vi "Node - Initial Handshaking.vi"(8 "error in (no error)":errorcluster, 11 "Node Data In":T1) -> (0 "error out":errorcluster, 3 "Node Data Out":T1)   [LabVIEW 2016, in "PXImc Router.lvlib"]
uses:
  PXImc Router.lvlib
  Controls/Node Data.ctl
  <vilib>/NI Veristand/VeriStand Data/Byte Buffer/Byte Buffer.lvclass
  Controls/Node/Node - PXImc Parameters.ctl
  Controls/Node/Transfer Data.ctl
  Controls/Node/Node Ch Properties.ctl
  Controls/Data Type.ctl
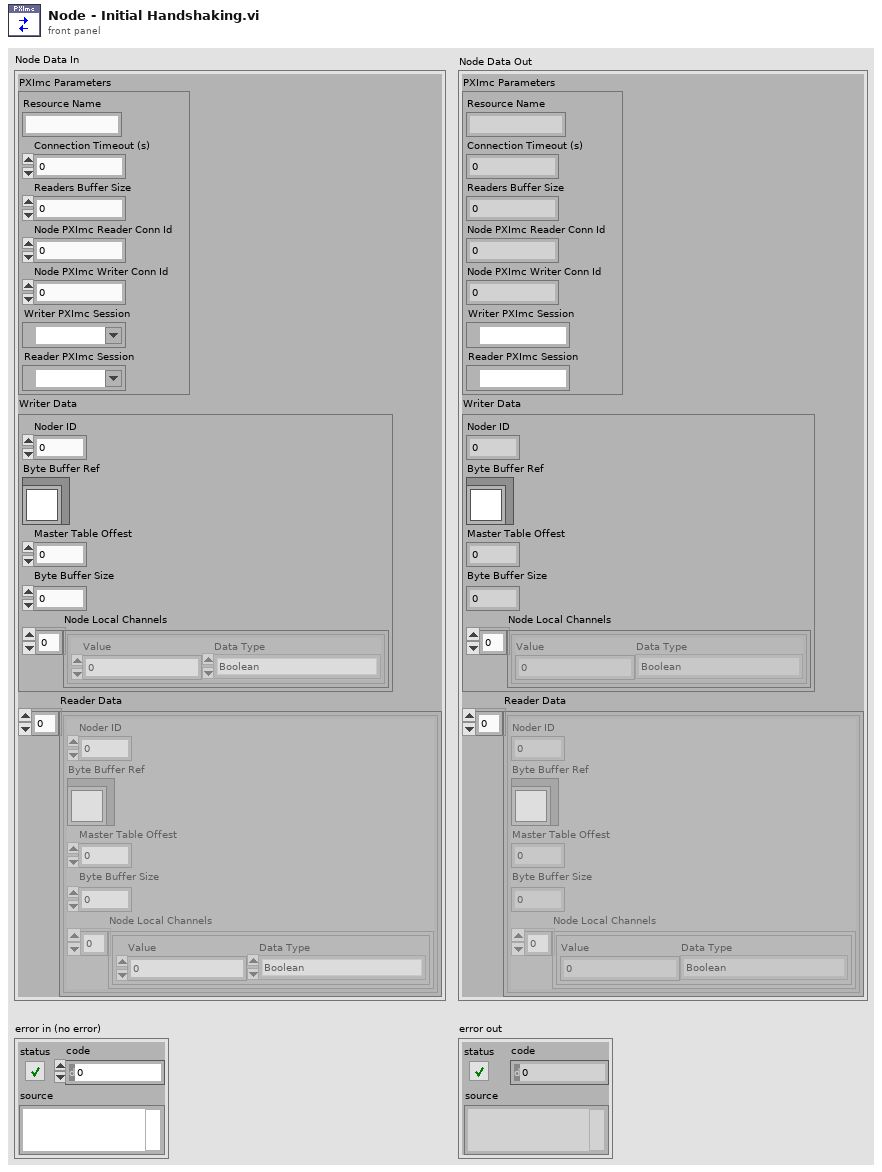
[diagram p1: front panel]
types:
  T1 = typedef "PXImc Router.lvlib/Node Data.ctl" = cluster{"PXImc Parameters":T2, "Writer Data":T3, "Reader Data":T3[]}
  T2 = typedef "PXImc Router.lvlib/Node - PXImc Parameters.ctl" = cluster{"Resource Name":string, "Connection Timeout (s)":dbl, "Readers Buffer Size":u64, "Node PXImc Reader Conn Id":u16, "Node PXImc Writer Conn Id":u16, "Writer PXImc Session":refnum<k21>, "Reader PXImc Session":refnum<k21>}
  T3 = typedef "PXImc Router.lvlib/Transfer Data.ctl" = cluster{"Noder ID":u32, "Byte Buffer Ref":refnum<class "Byte Buffer.lvclass">, "Master Table Offest":u32, "Byte Buffer Size":u32, "Node Local Channels":T4[]}
  T4 = typedef "PXImc Router.lvlib/Node Ch Properties.ctl" = cluster{"Value":dbl, "Data Type":T5}
  T5 = typedef "PXImc Router.lvlib/Data Type.ctl" = enum16{"Boolean", "SGL", "DBL", "I8", "I16", "I32", "I64", "U8", "U16", "U32", "U64"}
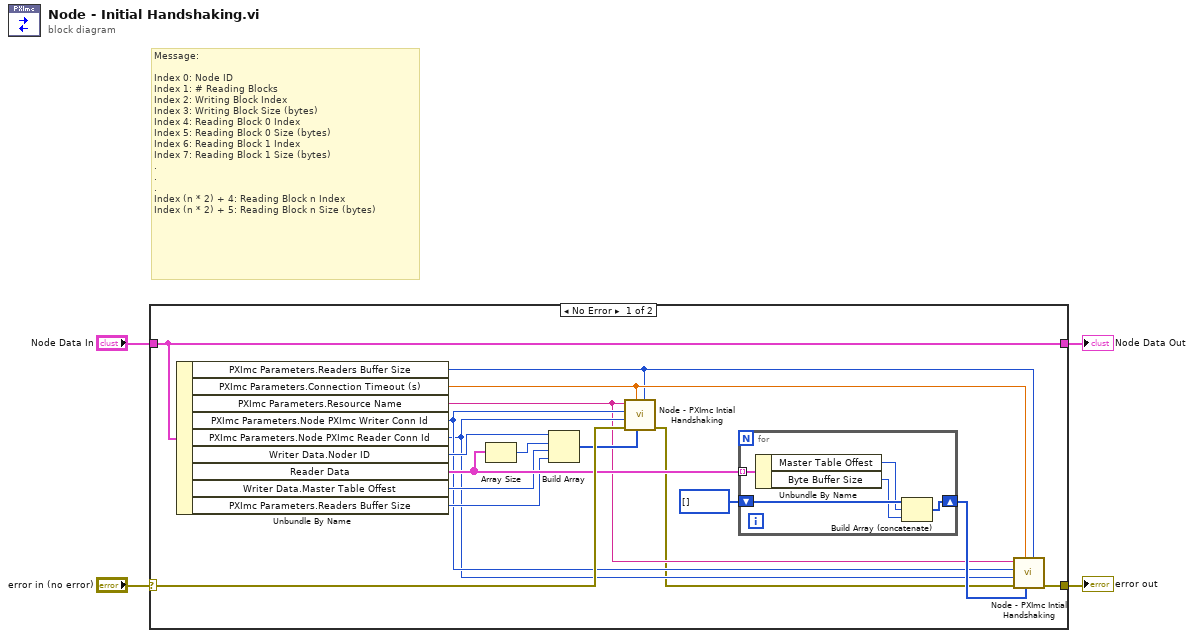
[diagram p0: block diagram]
diagram:
  # "Message:\n\nIndex 0: Node ID\nIndex 1: # Reading Blocks\nIndex 2: Writing Block Index\nIndex 3: Writing Block Size (bytes)\nIndex 4: Reading Block 0 Index\nIndex 5: Reading Block 0 Size (bytes)\nIndex 6: Reading Block 1 Index\nIndex 7: Reading Block 1 Size (bytes)\n.\n.\n.\nIndex (n * 2) + 4: Reading Block n Index\nIndex (n * 2) + 5: Reading Block n Size (bytes)"
  n1 = case shown="No Error" "error in (no error)" {
    selector: "error in (no error)" -> [w19 w28]
    tunnel: [w5 w28] -> w3
    tunnel: "Node Data In" -> [w21 w27]
    tunnel: [w21 w27] -> w1
    frame No Error {
      n2 = Unbundle By Name(w21) -> ("PXImc Parameters.Readers Buffer Size"=w10:u64, "PXImc Parameters.Connection Timeout (s)"=w11:dbl, "PXImc Parameters.Resource Name"=w7:string, "PXImc Parameters.Node PXImc Writer Conn Id"=w9:u16, "PXImc Parameters.Node PXImc Reader Conn Id"=w8:u16, "Writer Data.Noder ID"=w18:u32, "Reader Data"=w17:T3[], "Writer Data.Master Table Offest"=w15:u32, "PXImc Parameters.Readers Buffer Size"=w14:u64)
      n3 = Array Size(array=w17) -> (size(s)=w16:i32)
      n4 = Build Array(w18, w16, w15, w14) -> (w13:u64[])
      n5 = call "Node - PXImc Intial Handshaking.vi"("Reader Buffer Size In"=w10, "Data In"=w13, "Connection Timeout (s)"=w11, "error in (no error)"=w19, "Reader Conn ID"=w8, "Writer Conn ID"=w9, "Resource Name In"=w7) -> ("error out"=w6:errorcluster)  [unwired: 4 in]
      n6 = for {
        tunnel: w17 -> [w26] mode=indexing
        shift-right: [w22] -> w12
        shift-left: u32[] [] -> [w25]
        n7 = Unbundle By Name(w26) -> ("Master Table Offest"=w24:u32, "Byte Buffer Size"=w23:u32)
        n8 = Build Array (concatenate)(w25, w24, w23) -> (w22:u32[])
      }
      n9 = call "Node - PXImc Intial Handshaking.vi"("Reader Buffer Size In"=w10, "Data In"=w12, "Connection Timeout (s)"=w11, "error in (no error)"=w6, "Reader Conn ID"=w8, "Writer Conn ID"=w9, "Resource Name In"=w7) -> ("error out"=w5:errorcluster)  [unwired: 4 in]
    }
    frame Error {
    }
  }
  "Node Data Out" <- w1
  "error out" <- w3
